vi "NtfyLvFpga_SUB_SmtpSendMail.vi"(0 "smtp server":string, 1 "to[]":string[](array[string]), 2 "from":string, 3 "SMTP-AUTH":bool=TRUE, 5 "portNo(25)":i32=25, 7 "User-Id":string, 9 "password":string, 10 "Chk Server withSSL":bool, 11 "error in (no error)":errorcluster, 12 "subject":string="日本語のメール", 13 "body":string="日本語のメール", 14 "SSL":bool) -> (15 "error out":errorcluster)   [LabVIEW 2013]
uses:
  <vilib>/smtpClient/Set Message Text.vi
  <vilib>/smtpClient/LabVIEWSMTPClient.lvlib
  <vilib>/Utility/SMTP/NI_SMTPEmail.lvlib
panel:
  # "Send mail - by LabVIEW built-in E-Mail Function"
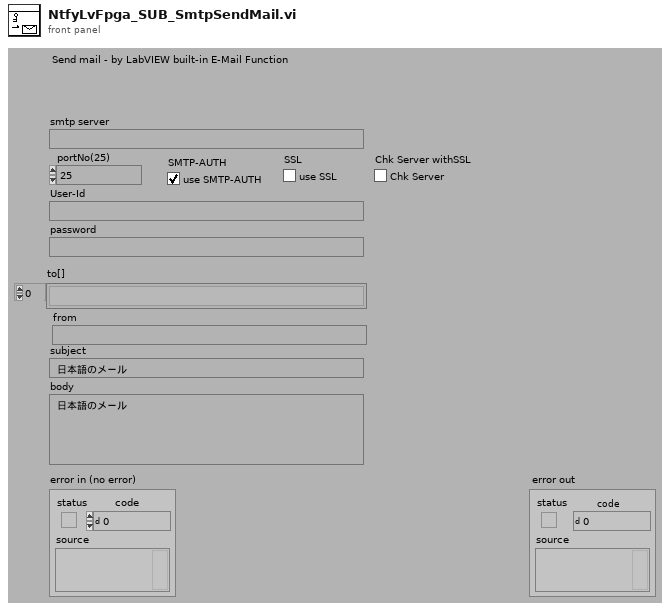
[diagram p1: front panel]
types:
  T1 = typedef "LabVIEWSMTPClient.lvlib/SmtpClientHandle.ctl" = refnum<k1>
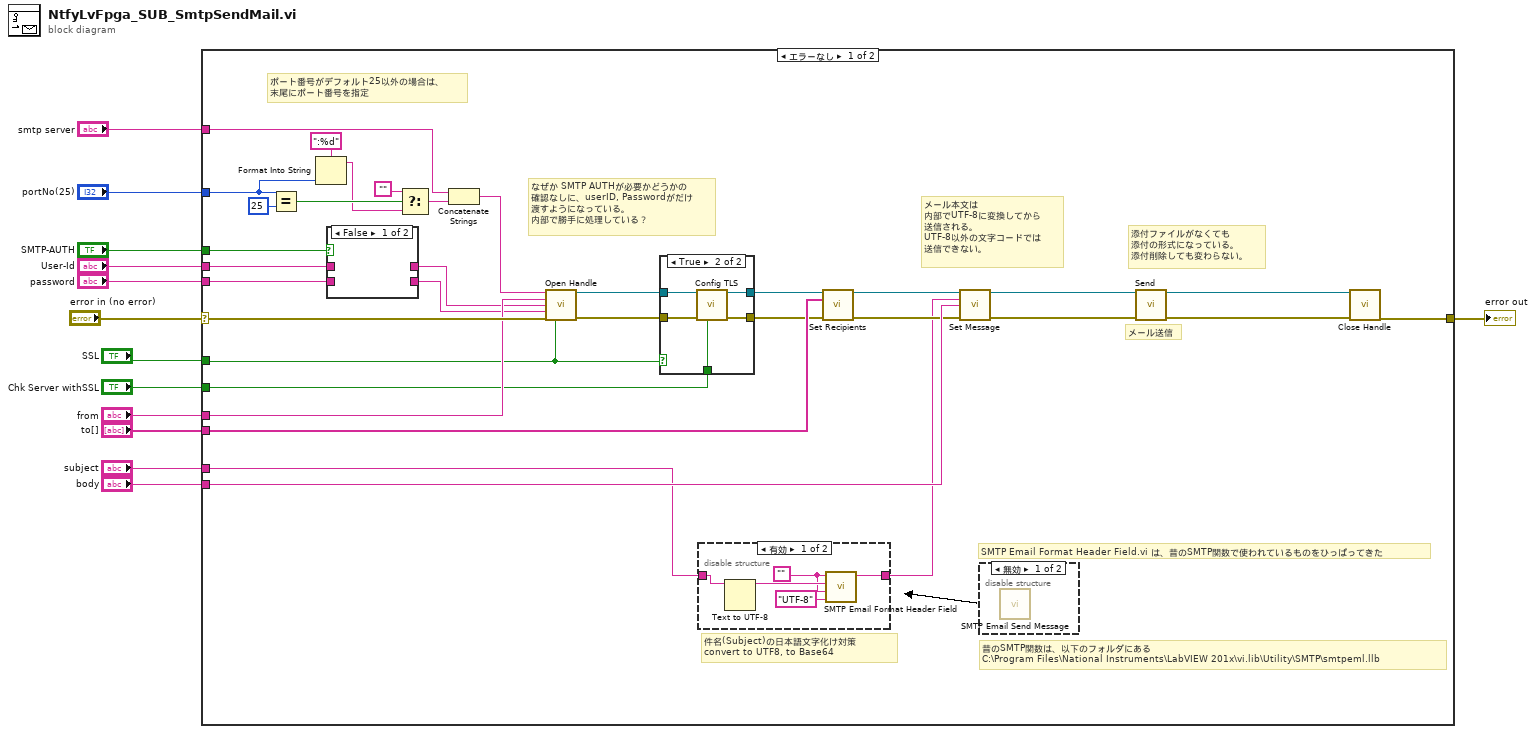
[diagram p0: block diagram]
diagram:
  n1 = case shown="エラーなし" "error in (no error)" {
    selector: "error in (no error)" -> [w46 w62]
    tunnel: [w21 w62] -> w4
    tunnel: "smtp server" -> [w25 _]
    tunnel: "portNo(25)" -> [w27 _]
    tunnel: "User-Id" -> [w17 _]
    tunnel: "password" -> [w16 _]
    tunnel: "to[]" -> [w38 _]
    tunnel: "from" -> [w39 _]
    tunnel: "subject" -> [w20 _]
    tunnel: "body" -> [w45 _]
    tunnel: "SSL" -> [w22 _]
    tunnel: "Chk Server withSSL" -> [w23 _]
    tunnel: "SMTP-AUTH" -> [w18 _]
    frame No Error {
      # "メール送信"
      # "添付ファイルがなくても\n添付の形式になっている。\n添付削除しても変わらない。"
      # "メール本文は\n内部でUTF-8に変換してから\n送信される。\nUTF-8以外の文字コードでは\n送信できない。"
      # "ポート番号がデフォルト25以外の場合は、\n末尾にポート番号を指定"
      # "SMTP Email Format Header Field.vi は、昔のSMTP関数で使われているものをひっぱってきた"
      # "昔のSMTP関数は、以下のフォルダにある\nC:\\Program Files\\National Instruments\\LabVIEW 201x\\vi.lib\\Utility\\SMTP\\smtpeml.llb"
      # "件名(Subject)の日本語文字化け対策\nconvert to UTF8, to Base64"
      # "なぜか SMTP AUTHが必要かどうかの\n確認なしに、userID, Passwordがだけ\n渡すようになっている。\n内部で勝手に処理している？"
      n2 = Equal?(x=w27, y=25) -> (x = y?=w31:bool)
      n3 = Format Into String(format string=":%d" ("形式文字列"), w27) -> (resulting string=w29:string)  [unwired: 2 in, 1 out]
      n4 = case shown="FALSE" w18 {
        tunnel: w17 -> [_ w48]
        tunnel: w16 -> [_ w47]
        tunnel: [_ w48] -> w15
        tunnel: [_ w47] -> w14
        frame False {
        }
        frame True {
        }
      }
      n5 = Select(t="", s=w31, f=w29) -> (s? t:f=w26:string)
      n6 = Concatenate Strings(w25, w26) -> (w24:string)
      n7 = call <vilib>:"Open Handle.vi"("server address"=w24, "from"=w39, "username"=w15, "password"=w14, "error in (no error)"=w46, "use TLS (false)"=w22) -> ("handle out"=w36:T1, "error out"=w34:errorcluster)  [unwired: 8 in]
      n8 = case shown="TRUE" w22 {
        tunnel: w36 -> [w56 w61]
        tunnel: [w56 w60] -> w35
        tunnel: w34 -> [w55 w59]
        tunnel: [w55 w58] -> w33
        tunnel: w23 -> [_ w57]
        frame False {
        }
        frame True {
          n9 = call <vilib>:"Config TLS.vi"("handle in"=w61, "error in (no error)"=w59, "verify server (true)"=w57) -> ("handle out"=w60:T1, "error out"=w58:errorcluster)  [unwired: 11 in]
        }
      }
      n10 = disable-structure shown="有効" {
        disable-tunnel: w20 -> [w53 w54]
        disable-tunnel: [w51 w54] -> w19
        frame Enabled {
          w50 = ""
          n11 = Text to UTF-8(11:w53) -> (3:w52:string)  [unwired: 1 in, 1 out]
          n12 = call <vilib>:"SMTP Email Format Header Field.vi"("character set"="UTF-8", "translit"=w50, "header content"=w52, "header name (Subject: )"=w50) -> ("encoded header line"=w51:string)  [unwired: 2 in, 1 out]
        }
        frame Disabled {
        }
      }
      n13 = call <vilib>:"Set Recipients.vi"("handle in"=w35, "to"=w38, "error in (no error)"=w33) -> ("handle out"=w40:T1, "error out"=w37:errorcluster)  [unwired: 11 in]
      n14 = call-poly <vilib>:"Set Message.vi"("handle in"=w40, "subject"=w19, "plain text message"=w45, "error in (no error)"=w37) -> ("handle out"=w44:T1, "error out"=w42:errorcluster)  [unwired: 10 in]
      n15 = disable-structure shown="無効" {
        frame Disabled {
          n16 = call <vilib>:"SMTP Email Send Message.vi"() -> ()  [unwired: 14 in, 2 out]
        }
        frame Enabled {
        }
      }
      n17 = call <vilib>:"Send.vi"("handle in"=w44, "error in (no error)"=w42) -> ("handle out"=w43:T1, "error out"=w41:errorcluster)  [unwired: 11 in, 1 out]
      n18 = call <vilib>:"Close Handle.vi"("handle in"=w43, "error in (no error)"=w41) -> ("error out"=w21:errorcluster)  [unwired: 12 in, 1 out]
    }
    frame Error {
    }
  }
  "error out" <- w4
